vi "_FPGA_PhaseDetector.vi"(1 "Reset":bool, 2 "Target":u32=1073741824, 3 "Cycle in":u64=4294967296) -> (0 "strobe out":bool)   [LabVIEW 2018]
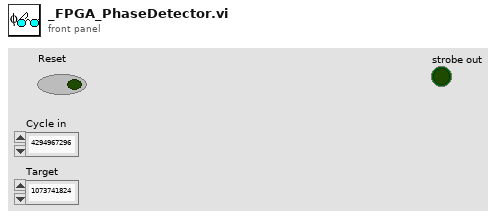
[diagram p1: front panel]
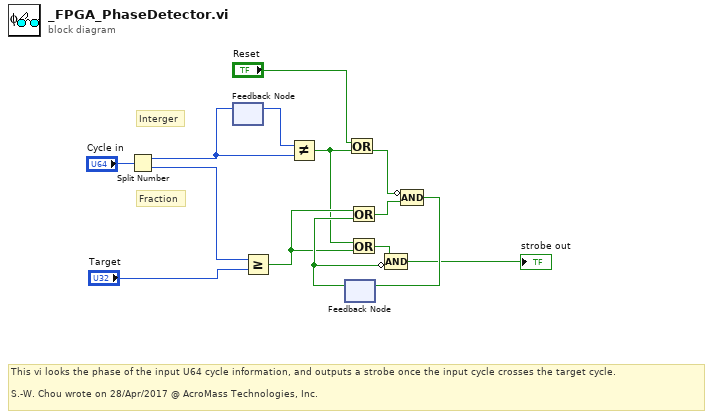
[diagram p0: block diagram]
diagram:
  # "This vi looks the phase of the input U64 cycle information, and outputs a strobe once the input cycle crosses the target cycle.\n\nS.-W. Chou wrote on 28/Apr/2017 @ AcroMass Technologies, Inc."
  # "Fraction"
  # "Interger"
  n1 = Split Number(x="Cycle in") -> (hi(x)=w8:u32, lo(x)=w11:u32)
  n2 = feedback-in #1(w8) -> ()
  n3 = feedback #1() -> (w12:u32)  [unwired: 1 in]
  n4 = Greater Or Equal?(x=w11, y="Target") -> (x >= y?=w6:bool)
  n5 = Not Equal?(x=w12, y=w8) -> (x != y?=w5:bool)
  n6 = feedback #2() -> (w7:bool)  [unwired: 1 in]
  n7 = Or(x="Reset", y=w5) -> (x .or. y?=w2:bool)
  n8 = Or(x=w6, y=w7) -> (x .or. y?=w10:bool)
  n9 = Or(x=w5, y=w6) -> (x .or. y?=w4:bool)
  n10 = Compound Arithmetic op=AND(w4, invert w7) -> (→"strobe out":bool)
  n11 = Compound Arithmetic op=AND(invert w2, w10) -> (w9:bool)
  n12 = feedback-in #2(w9) -> ()
